vi "DestroyRequestEvents.vi"(8 "error in (no error)":errorcluster) -> (0 "error out":errorcluster)   [LabVIEW 2018, in "AcPwrPlugins.lvlib"]
doc: "This VI destroys all the events that are used to broadcast messages to the Main.vi."
uses:
  AcPwrPlugins.lvlib
  AcPwrShared/AcPwrShared.lvlib
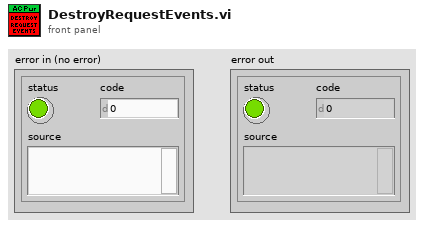
[diagram p1: front panel]
types:
  T1 = typedef "AcPwrShared.lvlib/clRequestEvents.ctl" = cluster{"StopRequest":refnum<user-event>, "PathToINI":refnum<user-event>, " LoadPlugin":refnum<user-event>, "ShowPanel":refnum<user-event>, "PrefDlg":refnum<user-event>, "InitAcPwr":refnum<user-event>, "Reset":refnum<user-event>, "Close":refnum<user-event>, "StopMeas":refnum<user-event>, "StartMeas":refnum<user-event>, "ConfigDevice":refnum<user-event>, "DeviceOn":refnum<user-event>, "DeviceOff":refnum<user-event>, "GetSettings":refnum<user-event>, "SetSettings":refnum<user-event>, "Abort":refnum<user-event>, "SetParameter":refnum<user-event>}
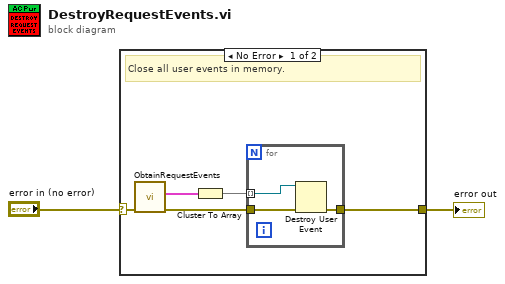
[diagram p0: block diagram]
diagram:
  n1 = case shown="No Error" "error in (no error)" {
    selector: "error in (no error)" -> [w6 w11]
    tunnel: [w5 w11] -> w1
    frame No Error {
      # "Close all user events in memory."
      n2 = call "ObtainRequestEvents.vi"("error in (no error)"=w6) -> ("error out"=w7:errorcluster, "AcPwrRequestEvents"=w4:T1)  [unwired: 9 in]
      n3 = Cluster To Array(cluster=w4) -> (array=w3:refnum<user-event>[])
      n4 = for {
        tunnel: w7 -> [w8]
        tunnel: [w10] -> w5
        tunnel: w3 -> [w9] mode=indexing
        n5 = Destroy User Event(user event=w9, error in=w8) -> (error out=w10:errorcluster)
      }
    }
    frame Error {
    }
  }
  "error out" <- w1
